vi "Save_MES_Data.vi"(9 "数组 2":string[](array[string]), 10 "XML文件路径":path[](array[path]), 11 "ListBox输入":refnum<vi>) -> (2 "数组":bool[](array[boolean]))   [LabVIEW 2018]
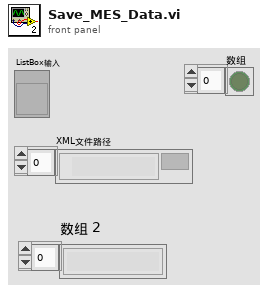
[diagram p1: front panel]
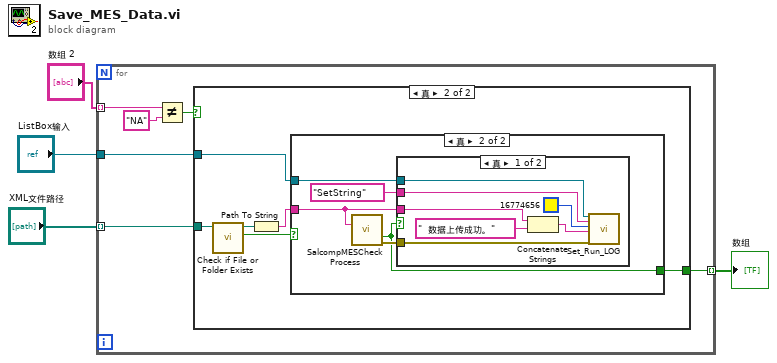
[diagram p0: block diagram]
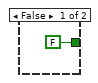
[diagram p2: hidden frame]
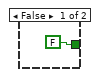
[diagram p3: hidden frame]
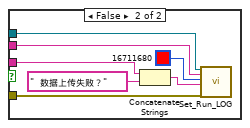
[diagram p4: hidden frame]
diagram:
  n1 = for {
    tunnel: "XML文件路径" -> [w9] mode=indexing
    tunnel: "ListBox输入" -> [w10]
    tunnel: [w8] -> w2 mode=indexing
    tunnel: "数组 2" -> [w7] mode=indexing
    n2 = Not Equal?(x=w7, y="NA") -> (x != y?=w6:bool)
    n3 = case shown="真" w6 {
      tunnel: w10 -> [_ w17]
      tunnel: w9 -> [_ w15]
      tunnel: [FALSE ("CheckRouteForSerialNumber") w12] -> w8
      frame False {
      }
      frame True {
        n4 = call <vilib>:"Check if File or Folder Exists.vi"("path"=w15) -> ("file or folder exists?"=w13:bool, "dup path"=w14:path)  [unwired: 8 in, 1 out]
        n5 = Path To String(path=w14) -> (string=w16:string)
        n6 = case shown="真" w13 {
          tunnel: w17 -> [_ w23]
          tunnel: w16 -> [_ w20]
          tunnel: [FALSE ("CheckRouteForSerialNumber") w19] -> w12
          frame False {
          }
          frame True {
            n7 = call "SalcompMESCheck Process.vi"("SN"=w20) -> ("CheckRouteForSerialNumber"=w19:bool, "错误输出"=w22:errorcluster)  [unwired: 12 in, 1 out]
            n8 = case shown="真" w19 {
              tunnel: w23 -> [w29 w36]
              tunnel: w22 -> [w28 w35]
              tunnel: "SetString" ("组合框") -> [w27 w34]
              tunnel: w20 -> [w25 w32]
              frame True {
                n9 = Concatenate Strings(w25, "  数据上传成功。") -> (w24:string)
                n10 = call "Set_Run_LOG.vi"("列表框 3"=w29, "组合框"=w27, "颜色盒"=u32 16774656, "字符串"=w24, "error in (no error)"=w28) -> ()  [unwired: 13 in, 2 out]
              }
              frame False {
                n11 = Concatenate Strings(w32, "  数据上传失败？") -> (w31:string)
                n12 = call "Set_Run_LOG.vi"("列表框 3"=w36, "组合框"=w34, "颜色盒"=u32 16711680, "字符串"=w31, "error in (no error)"=w35) -> ()  [unwired: 13 in, 2 out]
              }
            }
          }
        }
      }
    }
  }
  "数组" <- w2
